vi "NF90 calibrator.vi"(9 "Ports":T1, 10 "channel index":i8) -> ()   [LabVIEW 2015]
doc: "Illustrates the simplest form of TCP data acquisition using a TCP data server.\n\n\nCreated by Monroe Weber-Shirk\nCornell University\nmw24@cornell.edu\nJanuary 2000"
uses:
  NF90 move.ctl
  Axis.ctl
  DAC apps/support/method.ctl
  DataServer/command cluster.ctl
  DataServer/command.ctl
  DAQ configuration/Sensor array.ctl
  DAQ configuration/channel identifier.ctl
  NF90 commands.ctl
  DAQ configuration/Sensor buffer command.ctl
panel:
  in  "Go to Start":bool
  in  "Save Data":bool
  in  "Save Calibration":bool
  in  "Calibrate":bool
  in  "Go Home":bool
  in  "Done":bool
  in  "Find Home":bool
  in  "Acceleration":u8=6 min=1 max=50 step=1
  in  "Speed":sgl=1.0 min=0 max=3 format="%.3f"
  out "sample time":dbl format="%.2f"
  out "Sample rate":dbl format="%.2f"
  out "Error":cluster{sgl[], dbl[]}[](graph)
  in  "polynomial order":i32=2 min=1 max=5 step=1
  out "Calibation data":cluster{sgl[], "Best Polynomial Fit":dbl[]}[](graph)
  in  "Number of locations":u8=5 min=2 step=1
  in  "Start position":sgl min=-1048575 max=1048575 format="%.2f"
  in  "delay after move":u32=1000
  in  "Final position":sgl=10.0 min=-1048575 max=1048575 format="%.2f"
  in  "data points to acquire":u32=1000 min=1
  in  "method":T3={"sampling interval"=0.1, "samples to average"=1, "data interval"=0.0, "stream data"=FALSE, "file path"=refnum, "command"={"command"=enum."Idle", "start time (ms)"=0, "Channel Indices"=[], "Scans per Sample"=1}} {"command"."Scans per Sample" min=1; "data interval" format="%.2f"; "samples to average" min=1 step=1; "sampling interval" format="%.2f"}
  in  "move":T6={"axis"=enum."Z", "Increment"=0.0, "Speed"=1.0, "Acceleration"=1} {"Speed" min=0 format="%.3f"; "Acceleration" min=1 max=50 step=1; "Increment" format="%.3f"}
  in  "Home offset from limit switch":sgl min=-1048575 max=1048575 format="%.2f"
  out "Position":sgl(slide) min=0 max=6 step=-1 scale=0.0..1.0 scale format="%.2f"
  in  "serial port":refnum<visa-resource-name>="COM1"
  in  "stop":bool
  # "cm"
  # "cm/s"
  # "cm/s^2"
  # "cm"
  # "cm"
  # "Hz"
  # "s"
  # "ms"
  # "This code most likely doesn't work yet!"
  # "s"
  # "s"
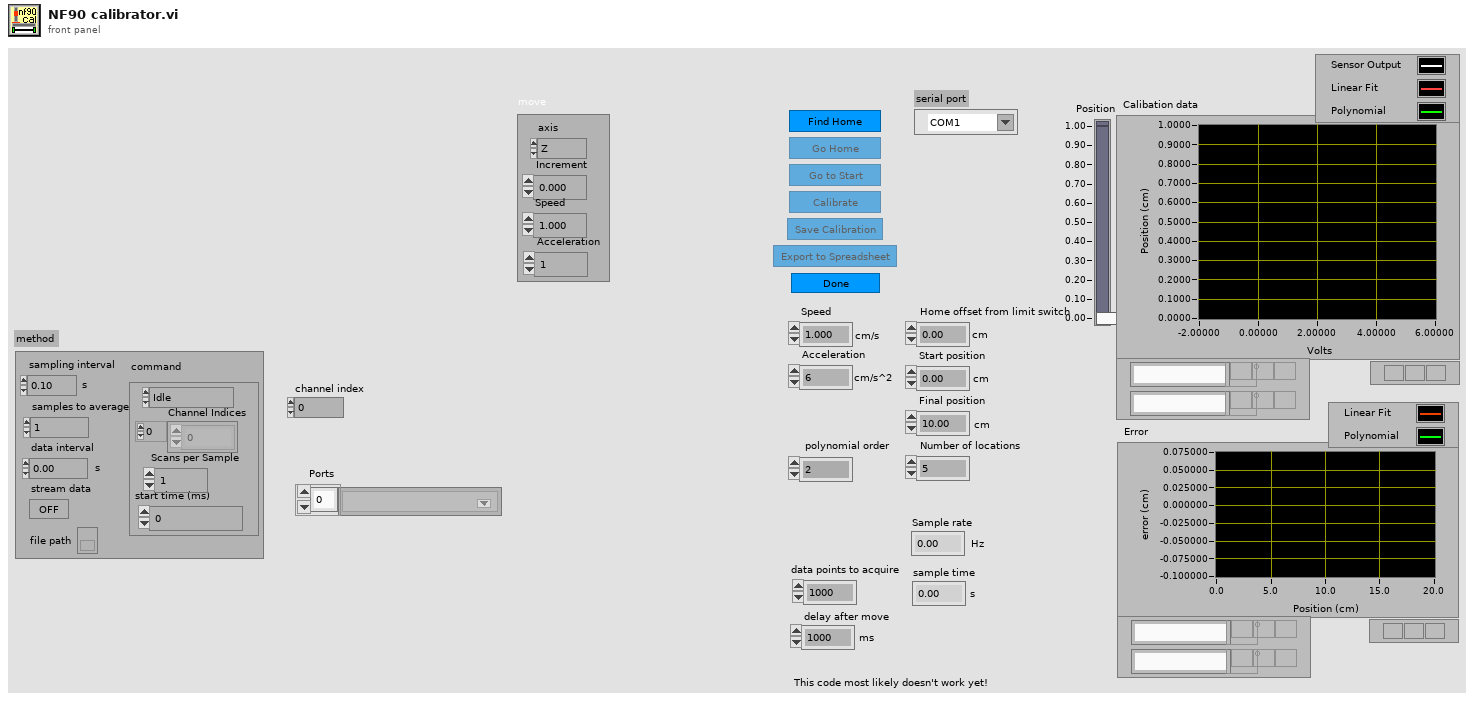
[diagram p1: front panel]
types:
  T1 = typedef "Sensor array.ctl" = T2[]
  T2 = typedef "channel identifier.ctl" = u16
  T3 = typedef "method.ctl" = cluster{"sampling interval":sgl, "samples to average":u32, "data interval":sgl, "stream data":bool, "file path":refnum<file>, "command":T4}
  T4 = typedef "command cluster.ctl" = cluster{"command":T5, "start time (ms)":u32, "Channel Indices":i32[], "Scans per Sample":i32}
  T5 = typedef "command.ctl" = enum16{"Idle", "Send Data", "Send 1 Scan", "Logoff"}
  T6 = typedef "NF90 move.ctl" = cluster{"axis":T7, "Increment":sgl, "Speed":sgl, "Acceleration":u8}
  T7 = typedef "Axis.ctl" = enum16{"X", "Y", "Z"}
  T8 = typedef "NF90 commands.ctl" = enum16{"Index", "Speed", "Acceleration", "Backlash", "Quit", "Run", "Null indexes", "Verify status", "Clear program", "Computer Control", "Go", "Put Controller on Hold", "Position"}
  T9 = typedef "Sensor buffer command.ctl" = enum16{"read average", "read recent", "read all", "write", "set buffer size", "Read channel config", "Write channel config", "clear"}
  T10 = typedef "Channel config.ctl" = cluster{"Channel Indices":T2[], "AI Max voltage":dbl[], "Calibration matrix":T11}
  T11 = typedef "calib array.ctl" = T12[]
  T12 = typedef "conversion.ctl" = cluster{"conversion matrix":sgl[][], "units":string, "name":string, "scale type":T13, "offset (volts)":dbl, "second channel":i8, "correspondence table":T14, "offset (physical units)":dbl, "pH scale":T15, "D.O.":T16, "Photometer data":T17}
  T13 = typedef "scale type.ctl" = enum16{"Volts", "Polynomial", "Correspondence Table", "pH", "Dissolved Oxygen", "Quadratic", "Photometer"}
  T14 = typedef "correspondence table.ctl" = cluster{"physical units":dbl, "volts":dbl}[]
  T15 = typedef "pH scale.ctl" = cluster{"Buffers":cluster{"Buffer":dbl, "Calibrated":bool, "V/T":dbl}[], "Temperature":dbl}
  T16 = typedef "DO scale.ctl" = cluster{"Temperature":dbl, "K":dbl, "barometric pressure":dbl}
  T17 = typedef "Photometer calibration data.ctl" = cluster{"Dark Voltage":dbl, "Blank Voltage":dbl, "Standards":cluster{"Concentration":dbl, "Voltage":dbl}[]}
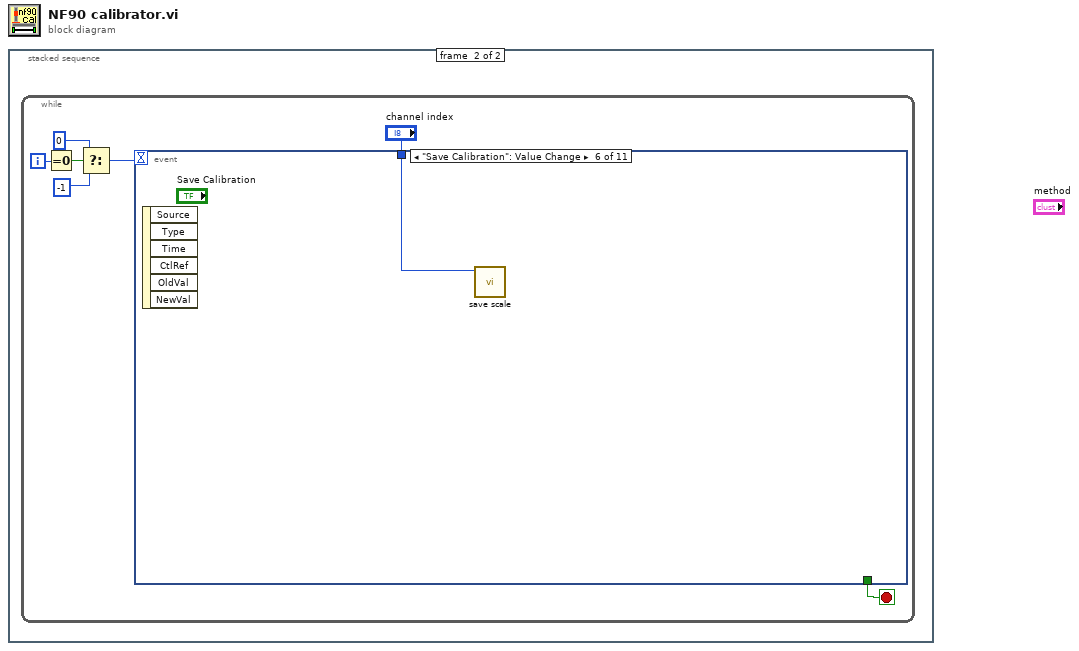
[diagram p0: block diagram]
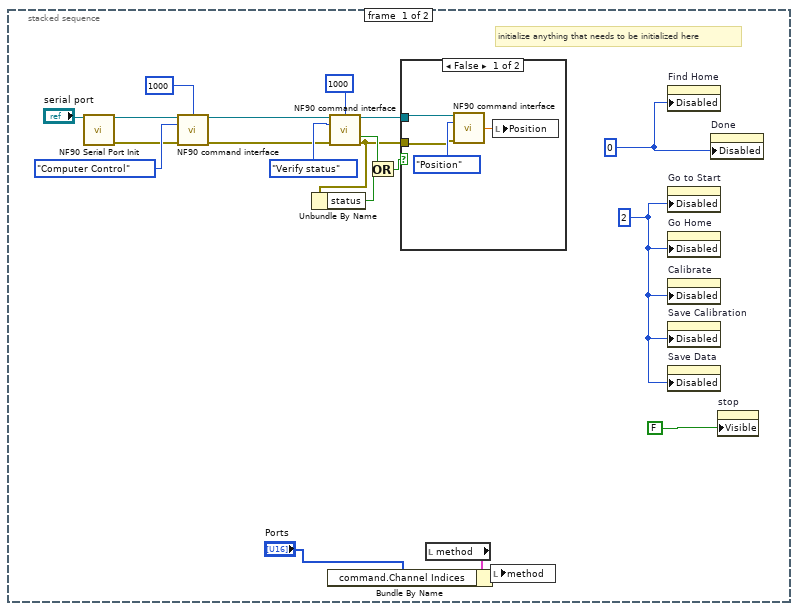
[diagram p2: hidden frame]
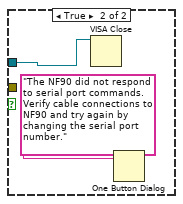
[diagram p3: hidden frame]
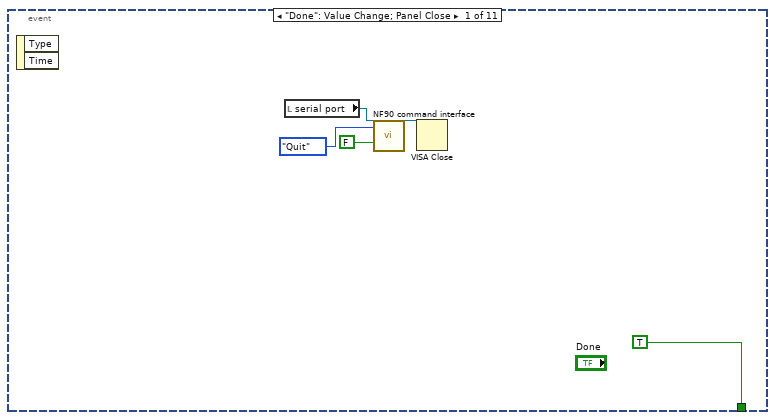
[diagram p4: hidden frame]
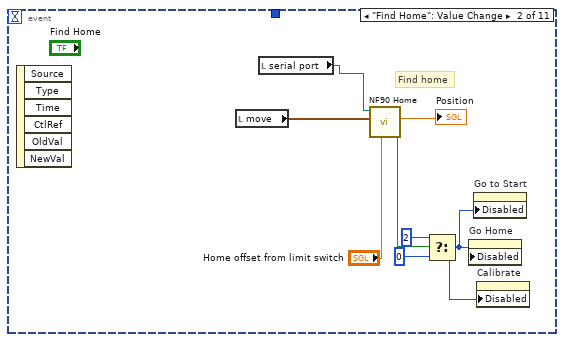
[diagram p5: hidden frame]
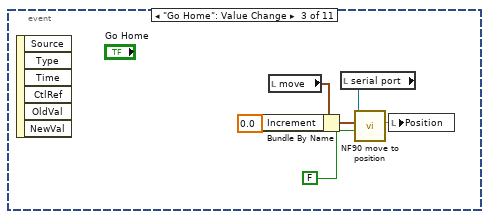
[diagram p6: hidden frame]
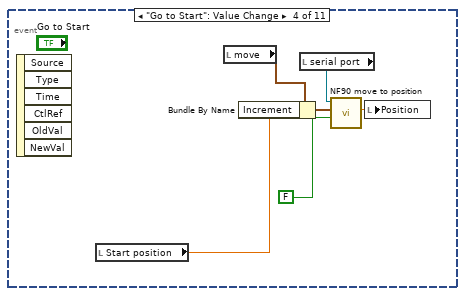
[diagram p7: hidden frame]
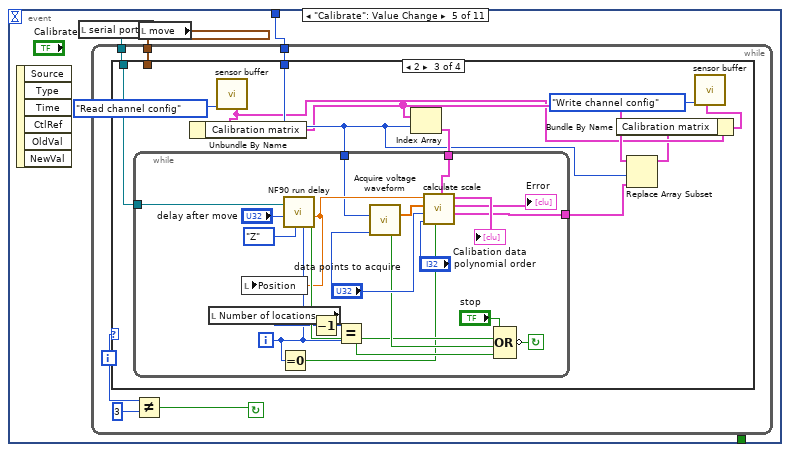
[diagram p8: hidden frame]
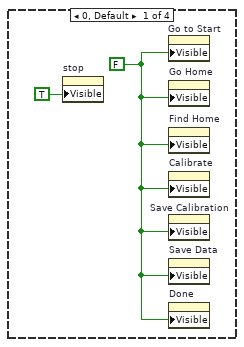
[diagram p9: hidden frame]
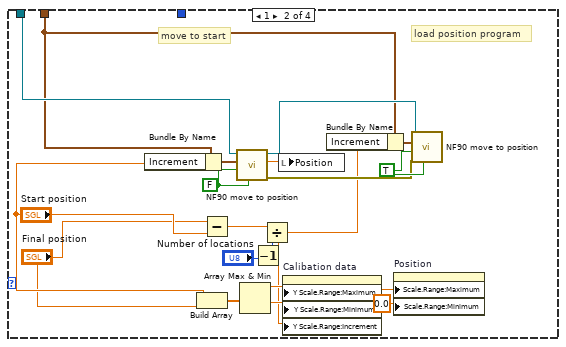
[diagram p10: hidden frame]
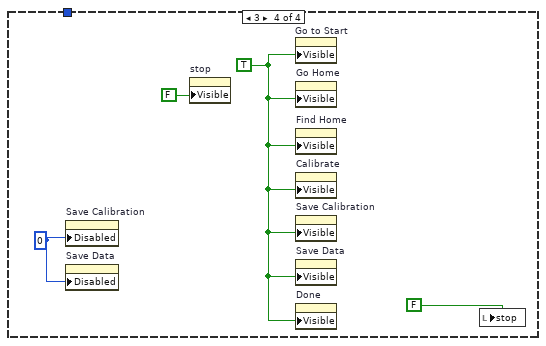
[diagram p11: hidden frame]
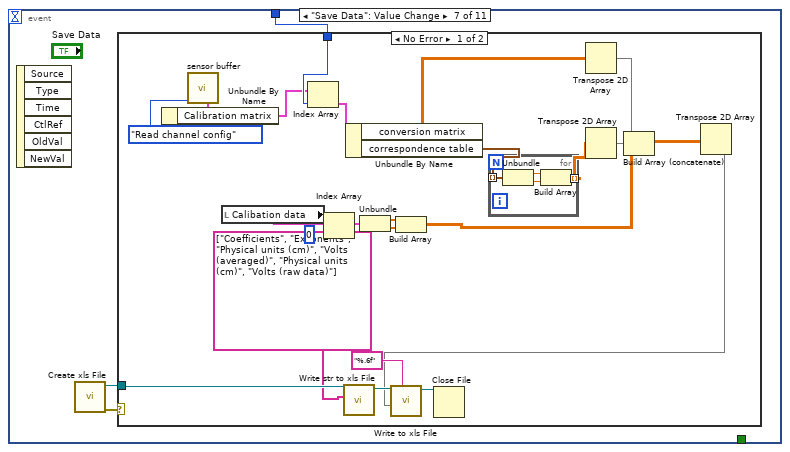
[diagram p12: hidden frame]
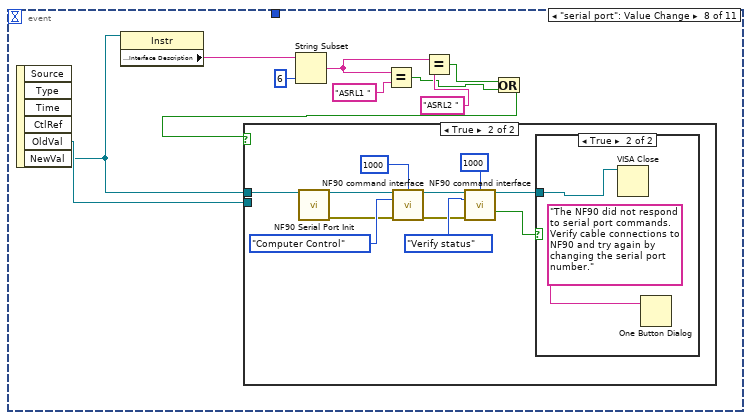
[diagram p14: hidden frame]
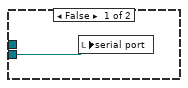
[diagram p15: hidden frame]
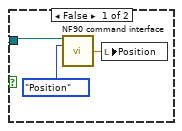
[diagram p16: hidden frame]
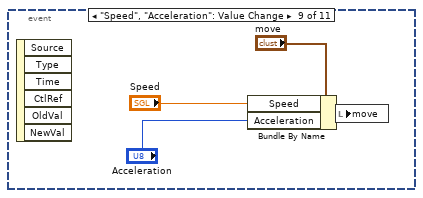
[diagram p17: hidden frame]
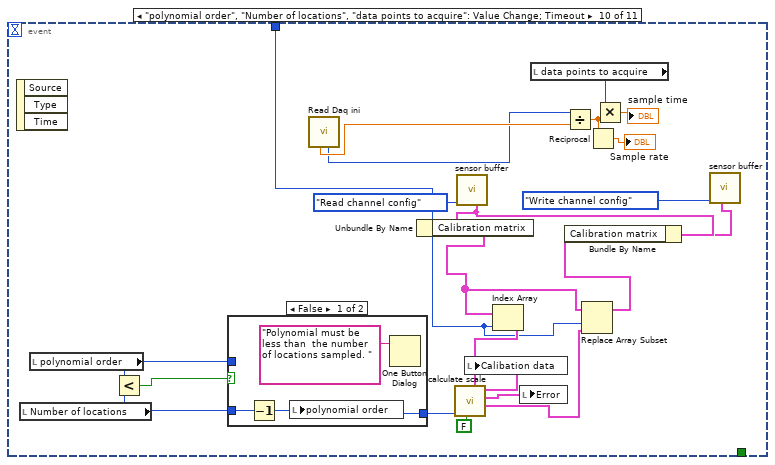
[diagram p18: hidden frame]
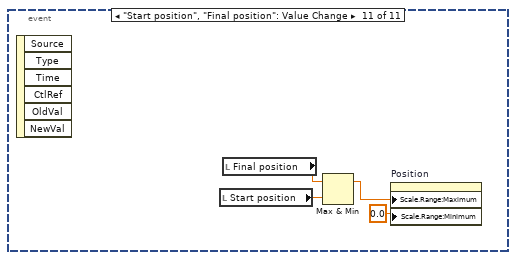
[diagram p20: hidden frame]
diagram:
  n1 = stacked-sequence {
    frame #0 {
      w10 = u8 2 ("Disabled")
      w9 = u8 0 ("Disabled")
      # "initialize anything that needs to be initialized here"
      n2 = call "NF90 Serial Port Init.vi"("port number"="serial port") -> ("port number"=w20:refnum<visa-resource-name>, "error out"=w7:errorcluster)  [unwired: 13 in]
      n3 = call "NF90 command interface.vi"("port number in"=w20, "time out (ms)"=u32 1000, "commands"=NF90_commands."Computer Control", "Error In"=w7) -> ("port number out"=w16:refnum<visa-resource-name>, "Error Out"=w6:errorcluster)  [unwired: 7 in, 3 out]
      n4 = call "NF90 command interface.vi"("port number in"=w16, "time out (ms)"=u32 1000, "commands"=NF90_commands."Verify status", "Error In"=w6) -> ("port number out"=w15:refnum<visa-resource-name>, "timed out"=w4:bool, "Error Out"=w2:errorcluster)  [unwired: 7 in, 2 out]
      n5 = Unbundle By Name(w2) -> ("status"=w5:bool)
      n6 = Or(x=w4, y=w5) -> (x .or. y?=w3:bool)
      n7 = case shown="False" w3 {
        tunnel: w15 -> [w22 w25]
        tunnel: w2 -> [w21 _]
        frame False {
          n8 = call "NF90 command interface.vi"("port number in"=w22, "commands"=NF90_commands."Position", "Error In"=w21) -> ("Position"=w23:sgl)  [unwired: 8 in, 4 out]
          n9 = local write "Position"(w23) -> ()
        }
        frame True {
          n10 = VISA Close(VISA resource name=w25) -> ()  [unwired: 1 in, 1 out]
          n11 = One Button Dialog(message="The NF90 did not respond to serial port commands. Verify cable connections to NF90 and try again by changing the serial port number.") -> ()  [unwired: 1 in, 1 out]
        }
      }
      n12 = local read "method"() -> (w12:T3)
      n13 = Bundle By Name(cluster=w12, "command.Channel Indices"="Ports") -> (w11:T3)
      n14 = local write "method"(w11) -> ()
      n15 = property on="Find Home" class="Bool"("Disabled"=w9) -> ()  [unwired: 2 in, 2 out]
      n16 = property on="Go to Start" class="Bool"("Disabled"=w10) -> ()  [unwired: 2 in, 2 out]
      n17 = property on="Go Home" class="Bool"("Disabled"=w10) -> ()  [unwired: 2 in, 2 out]
      n18 = property on="Calibrate" class="Bool"("Disabled"=w10) -> ()  [unwired: 2 in, 2 out]
      n19 = property on="Save Calibration" class="Bool"("Disabled"=w10) -> ()  [unwired: 2 in, 2 out]
      n20 = property on="Save Data" class="Bool"("Disabled"=w10) -> ()  [unwired: 2 in, 2 out]
      n21 = property on="Done" class="Bool"("Disabled"=w9) -> ()  [unwired: 2 in, 2 out]
      n22 = property on="stop" class="Bool (strict)"("Visible"=FALSE) -> ()  [unwired: 2 in, 2 out]
    }
    frame #1 {
      n23 = while {
        i -> [w31]
        stop <- w32 stop-if-true
        n24 = Equal To 0?(x=w31) -> (x = 0?=w30:bool)
        n25 = Select(t=0, s=w30, f=-1) -> (s? t:f=w27:i32)
        n26 = event shown="[5] \"Save Calibration\": Value Change" {
          selector: _ -> [_ _ _ _ _ _ _ _ _ _ _]
          dyn-events: _ -> [_ _ _ _ _ _ _ _ _ _ _]
          timeout: w27 -> [_ _ _ _ _ _ _ _ _ _ _]
          tunnel: "channel index" -> [_ _ _ _ w61 w124 w125 _ _ w194 _]
          tunnel: [TRUE _ _ _ _ _ _ _ _ _ _] -> w32
          event "Done": Value Change; Panel Close {
            n27 = event-data() -> ()  [unwired: 1 in, 2 out]
            n28 = local read "serial port"() -> (w35:refnum<visa-resource-name>)
            n29 = call "NF90 command interface.vi"("port number in"=w35, "commands"=NF90_commands."Quit", "enable?"=FALSE) -> ("port number out"=w38:refnum<visa-resource-name>)  [unwired: 8 in, 4 out]
            n30 = VISA Close(VISA resource name=w38) -> ()  [unwired: 1 in, 1 out]
          }
          event "Find Home": Value Change {
            # "Find home"
            n31 = event-data() -> ()  [unwired: 1 in, 6 out]
            n32 = local read "move"() -> (w41:T6)
            n33 = local read "serial port"() -> (w40:refnum<visa-resource-name>)
            n34 = call "NF90 Home.vi"("Index offset from switch"="Home offset from limit switch", "move"=w41, "port number in"=w40) -> ("killed"=w44:bool, "position"=→"Position":dbl)  [unwired: 4 in, 2 out]
            n35 = Select(t=2, s=w44, f=0) -> (s? t:f=w39:i32)
            n36 = property on="Go Home" class="Bool"("Disabled"=w39) -> ()  [unwired: 2 in, 2 out]
            n37 = property on="Go to Start" class="Bool"("Disabled"=w39) -> ()  [unwired: 2 in, 2 out]
            n38 = property on="Calibrate" class="Bool"("Disabled"=w39) -> ()  [unwired: 2 in, 2 out]
          }
          event "Go Home": Value Change {
            n39 = event-data() -> ()  [unwired: 1 in, 6 out]
            n40 = local read "move"() -> (w47:T6)
            n41 = Bundle By Name(cluster=w47, "Increment"=sgl 0.0 ("Bundle Element")) -> (w49:T6)
            n42 = local read "serial port"() -> (w48:refnum<visa-resource-name>)
            n43 = call "NF90 move to position.vi"("move type (abs = False)"=FALSE ("move type (abs = true)"), "move"=w49, "port number in"=w48) -> ("Position out"=w52:sgl)  [unwired: 4 in, 3 out]
            n44 = local write "Position"(w52) -> ()
          }
          event "Go to Start": Value Change {
            n45 = event-data() -> ()  [unwired: 1 in, 6 out]
            n46 = local read "Start position"() -> (w58:sgl)
            n47 = local read "move"() -> (w53:T6)
            n48 = Bundle By Name(cluster=w53, "Increment"=w58) -> (w55:T6)
            n49 = local read "serial port"() -> (w54:refnum<visa-resource-name>)
            n50 = call "NF90 move to position.vi"("move type (abs = False)"=FALSE ("move type (abs = true)"), "move"=w55, "port number in"=w54) -> ("Position out"=w57:sgl)  [unwired: 4 in, 3 out]
            n51 = local write "Position"(w57) -> ()
          }
          event "Calibrate": Value Change {
            n52 = event-data() -> ()  [unwired: 1 in, 6 out]
            n53 = local read "serial port"() -> (w60:refnum<visa-resource-name>)
            n54 = local read "move"() -> (w59:T6)
            n55 = while {
              tunnel: w60 -> [w65]
              tunnel: w59 -> [w66]
              tunnel: w61 -> [w62]
              i -> [w67]
              stop <- w63 continue-if-true
              n56 = case shown="2" w67 {
                tunnel: w66 -> [_ w81 _ _]
                tunnel: w65 -> [_ w87 w98 _]
                tunnel: w62 -> [_ _ w95 _]
                frame 0, Default {
                  w69 = FALSE ("Visible")
                  n57 = property on="stop" class="Bool (strict)"("Visible"=TRUE) -> ()  [unwired: 2 in, 2 out]
                  n58 = property on="Go to Start" class="Bool"("Visible"=w69) -> ()  [unwired: 2 in, 2 out]
                  n59 = property on="Go Home" class="Bool"("Visible"=w69) -> ()  [unwired: 2 in, 2 out]
                  n60 = property on="Find Home" class="Bool"("Visible"=w69) -> ()  [unwired: 2 in, 2 out]
                  n61 = property on="Calibrate" class="Bool"("Visible"=w69) -> ()  [unwired: 2 in, 2 out]
                  n62 = property on="Save Calibration" class="Bool"("Visible"=w69) -> ()  [unwired: 2 in, 2 out]
                  n63 = property on="Save Data" class="Bool"("Visible"=w69) -> ()  [unwired: 2 in, 2 out]
                  n64 = property on="Done" class="Bool"("Visible"=w69) -> ()  [unwired: 2 in, 2 out]
                }
                frame 1 {
                  w80 = FALSE ("move type (abs = true)")
                  w79 = TRUE ("move type (abs = False)")
                  # "move to start"
                  # "load position program"
                  n65 = Bundle By Name(cluster=w81, "Increment"="Start position") -> (w88:T6)
                  n66 = Build Array("Start position", "Final position") -> (w74:sgl[])
                  n67 = Subtract(x="Final position", y="Start position") -> (x-y=w84:sgl)
                  n68 = call "NF90 move to position.vi"("program (Run=False)"=w80, "move type (abs = False)"=w80, "move"=w88, "port number in"=w87) -> ("Error Out"=w78:errorcluster, "Position out"=w77:sgl, "port number out"=w86:refnum<visa-resource-name>)  [unwired: 3 in, 1 out]
                  n69 = Array Max & Min(array=w74) -> (max value=w73:sgl, min value=w72:sgl)  [unwired: 2 out]
                  n70 = Decrement(x="Number of locations") -> (x-1=w83:u8)
                  n71 = Divide(x=w84, y=w83) -> (x/y=w71:sgl)
                  n72 = local write "Position"(w77) -> ()
                  n73 = property on="Calibation data" class="XYGraph (strict)"("Y Scale.Range:Maximum"=w73, "Y Scale.Range:Minimum"=w72, "Y Scale.Range:Increment"=w71) -> ()  [unwired: 2 in, 2 out]
                  n74 = Bundle By Name(cluster=w81, "Increment"=w71) -> (w82:T6)
                  n75 = property on="Position" class="Slide (strict)"("Scale.Range:Maximum"=w73, "Scale.Range:Minimum"=0.0) -> ()  [unwired: 2 in, 2 out]
                  n76 = call "NF90 move to position.vi"("program (Run=False)"=w79, "Error In"=w78, "move type (abs = False)"=w79, "move"=w82, "port number in"=w86) -> ()  [unwired: 2 in, 4 out]
                }
                frame 2 {
                  n77 = call "sensor buffer.vi"("command"=Sensor_buffer_command."Read channel config") -> ("Channel Config out"=w91:T10)  [unwired: 6 in, 4 out]
                  n78 = Unbundle By Name(w91) -> ("Calibration matrix"=w93:T11)
                  n79 = Index Array(array=w93, index=w95) -> (element=w97:T12)
                  n80 = while {
                    tunnel: [w106] -> w96
                    tunnel: w98 -> [w119]
                    tunnel: w95 -> [w100]
                    tunnel: w97 -> [w99]
                    i -> [w102]
                    stop <- w116 continue-if-true
                    n81 = local read "Number of locations"() -> (w112:u8)
                    n82 = Equal To 0?(x=w102) -> (x = 0?=w101:bool)
                    n83 = call "NF90 run delay.vi"("i"=w102, "axis"=Axis."Z", "delay (ms)"="delay after move", "port number"=w119) -> ("Position"=w108:sgl, "killed"=w114:bool)  [unwired: 4 in, 2 out]
                    n84 = local write "Position"(w108) -> ()
                    n85 = Decrement(x=w112) -> (x-1=w105:u8)
                    n86 = Equal?(x=w105, y=w102) -> (x = y?=w111:bool)
                    n87 = call "Acquire voltage waveform.vi"("channel index"=w100, "data points to acquire"="data points to acquire") -> ("channel data array"=w109:sgl[], "canceled"=w115:bool)  [unwired: 10 in, 2 out]
                    n88 = call "calculate scale.vi"("Scaling in"=w99, "reset"=w101, "polynomial order"="polynomial order", "data points to acquire"="data points to acquire", "volts array"=w109, "Position"=w108) -> ("Scaling out"=w106:T12, "error graph"=→"Error":cluster{"X array":sgl[], "Y array":dbl[]}[], "Output Graph"=→"Calibation data":cluster{"X array":sgl[], "Y array":dbl[]}[])  [unwired: 2 in]
                    n89 = Compound Arithmetic op=OR("stop", w114, w115, w111) -> (invert w116:bool)
                  }
                  n90 = Replace Array Subset(array=w93, new element=w96, index=w95) -> (w89:T11)
                  n91 = Bundle By Name(cluster=w91, "Calibration matrix"=w89) -> (w90:T10)
                  n92 = call "sensor buffer.vi"("Channel Config"=w90, "command"=Sensor_buffer_command."Write channel config") -> ()  [unwired: 5 in, 5 out]
                }
                frame 3 {
                  w122 = TRUE ("Visible")
                  w120 = u8 0 ("Disabled")
                  n93 = property on="Save Calibration" class="Bool"("Disabled"=w120) -> ()  [unwired: 2 in, 2 out]
                  n94 = property on="Save Data" class="Bool"("Disabled"=w120) -> ()  [unwired: 2 in, 2 out]
                  n95 = property on="stop" class="Bool (strict)"("Visible"=FALSE) -> ()  [unwired: 2 in, 2 out]
                  n96 = property on="Go to Start" class="Bool"("Visible"=w122) -> ()  [unwired: 2 in, 2 out]
                  n97 = property on="Go Home" class="Bool"("Visible"=w122) -> ()  [unwired: 2 in, 2 out]
                  n98 = property on="Find Home" class="Bool"("Visible"=w122) -> ()  [unwired: 2 in, 2 out]
                  n99 = property on="Calibrate" class="Bool"("Visible"=w122) -> ()  [unwired: 2 in, 2 out]
                  n100 = property on="Save Calibration" class="Bool"("Visible"=w122) -> ()  [unwired: 2 in, 2 out]
                  n101 = property on="Save Data" class="Bool"("Visible"=w122) -> ()  [unwired: 2 in, 2 out]
                  n102 = property on="Done" class="Bool"("Visible"=w122) -> ()  [unwired: 2 in, 2 out]
                  n103 = local write "stop"(FALSE ("Visible")) -> ()
                }
              }
              n104 = Not Equal?(x=w67, y=3) -> (x != y?=w63:bool)
            }
          }
          event "Save Calibration": Value Change {
            n105 = event-data() -> ()  [unwired: 1 in, 6 out]
            n106 = call "save scale.vi"("Index"=w124) -> ()  [unwired: 9 in, 1 out]
          }
          event "Save Data": Value Change {
            n107 = event-data() -> ()  [unwired: 1 in, 6 out]
            n108 = call "Create xls File.vi"() -> ("error out"=w127:errorcluster, "refnum"=w126:refnum<file>)  [unwired: 4 in, 2 out]
            n109 = case shown="No Error" w127 {
              tunnel: w126 -> [w134 _]
              tunnel: w125 -> [w133 _]
              frame No Error {
                n110 = call "sensor buffer.vi"("command"=Sensor_buffer_command."Read channel config") -> ("Channel Config out"=w129:T10)  [unwired: 6 in, 4 out]
                n111 = Unbundle By Name(w129) -> ("Calibration matrix"=w128:T11)
                n112 = local read "Calibation data"() -> (w138:cluster{sgl[], "Best Polynomial Fit":dbl[]}[])
                n113 = Index Array(array=w128, index=w133) -> (element=w132:T12)
                n114 = Index Array(array=w138, index=0 ("Index")) -> (element=w137:cluster{sgl[], "Best Polynomial Fit":dbl[]})
                n115 = call "Write str to xls File.vi"("1D data"=string[] ["Coefficients", "Exponents", "Physical units (cm)", "Volts (averaged)", "Physical units (cm)", "Volts (raw data)"], "refnum"=w134) -> ("dup refnum"=w150:refnum<file>)  [unwired: 8 in, 1 out]
                n116 = Unbundle By Name(w132) -> ("conversion matrix"=w145:sgl[][], "correspondence table"=w148:T14)
                n117 = Unbundle(w137) -> (w140:sgl[], "Best Polynomial Fit"=w139:dbl[])
                n118 = Build Array(w140, w139) -> (w135:dbl[][])
                n119 = for {
                  tunnel: w148 -> [w154] mode=indexing
                  tunnel: [w151] -> w147 mode=indexing
                  n120 = Unbundle(w154) -> ("physical units"=w153:dbl, "volts"=w152:dbl)
                  n121 = Build Array(w153, w152) -> (w151:dbl[])
                }
                n122 = Transpose 2D Array(2D array=w145) -> (transposed array=w143:sgl[][])
                n123 = Transpose 2D Array(2D array=w147) -> (transposed array=w142:dbl[][])
                n124 = Build Array (concatenate)(w143, w142, w135) -> (w146:dbl[][])
                n125 = Transpose 2D Array(2D array=w146) -> (transposed array=w141:dbl[][])
                n126 = call "Write to xls File.vi"("format (%.3f)"="%.6f", "2D data"=w141, "refnum"=w150) -> ("dup refnum"=w149:refnum<file>)  [unwired: 7 in, 1 out]
                n127 = Close File(refnum=w149) -> ()  [unwired: 1 in, 2 out]
              }
              frame Error {
              }
            }
          }
          event "serial port": Value Change {
            n128 = event-data() -> ("OldVal"=w163:refnum<visa-resource-name>, "NewVal"=w155:refnum<visa-resource-name>)  [unwired: 1 in, 4 out]
            n129 = property class="Instr"(reference=w155) -> ("Interface Information:Interface Description"=w158:string)  [unwired: 1 in, 2 out]
            n130 = String Subset(string=w158, length (rest)=6 ("length (rest)")) -> (substring=w157:string)  [unwired: 1 in]
            n131 = Equal?(x=w157, y="ASRL1 ") -> (x = y?=w160:bool)
            n132 = Equal?(x=w157, y="ASRL2 ") -> (x = y?=w161:bool)
            n133 = Or(x=w161, y=w160) -> (x .or. y?=w159:bool)
            n134 = case shown="True" w159 {
              tunnel: w155 -> [_ w166]
              tunnel: w163 -> [w165 _]
              frame False {
                n135 = local write "serial port"(w165) -> ()
              }
              frame True {
                n136 = call "NF90 Serial Port Init.vi"("port number"=w166) -> ("port number"=w176:refnum<visa-resource-name>, "error out"=w168:errorcluster)  [unwired: 13 in]
                n137 = call "NF90 command interface.vi"("port number in"=w176, "time out (ms)"=u32 1000, "commands"=NF90_commands."Computer Control", "Error In"=w168) -> ("port number out"=w173:refnum<visa-resource-name>, "Error Out"=w167:errorcluster)  [unwired: 7 in, 3 out]
                n138 = call "NF90 command interface.vi"("port number in"=w173, "time out (ms)"=u32 1000, "commands"=NF90_commands."Verify status", "Error In"=w167) -> ("port number out"=w172:refnum<visa-resource-name>, "timed out"=w169:bool)  [unwired: 7 in, 3 out]
                n139 = case shown="True" w169 {
                  tunnel: w172 -> [w177 w180]
                  frame False {
                    n140 = call "NF90 command interface.vi"("port number in"=w177, "commands"=NF90_commands."Position") -> ("Position"=w178:sgl)  [unwired: 9 in, 4 out]
                    n141 = local write "Position"(w178) -> ()
                  }
                  frame True {
                    n142 = VISA Close(VISA resource name=w180) -> ()  [unwired: 1 in, 1 out]
                    n143 = One Button Dialog(message="The NF90 did not respond to serial port commands. Verify cable connections to NF90 and try again by changing the serial port number.") -> ()  [unwired: 1 in, 1 out]
                  }
                }
              }
            }
          }
          event "Speed", "Acceleration": Value Change {
            n144 = event-data() -> ()  [unwired: 1 in, 6 out]
            n145 = Bundle By Name(cluster="move", "Speed"="Speed", "Acceleration"="Acceleration") -> (w182:T6)
            n146 = local write "move"(w182) -> ()
          }
          event "polynomial order", "Number of locations", "data points to acquire": Value Change; Timeout {
            n147 = event-data() -> ()  [unwired: 1 in, 3 out]
            n148 = local read "Number of locations"() -> (w197:u8)
            n149 = local read "polynomial order"() -> (w195:i32)
            n150 = Less?(x=w195, y=w197) -> (x < y?=w196:bool)
            n151 = case shown="False" w196 {
              tunnel: w197 -> [w210 _]
              tunnel: [w208 w211] -> w198
              tunnel: w195 -> [_ w211]
              frame False {
                n152 = Decrement(x=w210) -> (x-1=w208:u8)
                n153 = local write "polynomial order"(w208) -> ()
                n154 = One Button Dialog(message="Polynomial must be less than  the number of locations sampled. ") -> ()  [unwired: 1 in, 1 out]
              }
              frame True {
              }
            }
            n155 = call "Read Daq ini.vi"() -> ("samples per read"=w186:i32, "Data rate (hz)"=w187:dbl)  [unwired: 3 in, 7 out]
            n156 = call "sensor buffer.vi"("command"=Sensor_buffer_command."Read channel config") -> ("Channel Config out"=w189:T10)  [unwired: 6 in, 4 out]
            n157 = Unbundle By Name(w189) -> ("Calibration matrix"=w191:T11)
            n158 = Index Array(array=w191, index=w194) -> (element=w202:T12)
            n159 = call "calculate scale.vi"("Scaling in"=w202, "reset"=FALSE, "polynomial order"=w198) -> ("Scaling out"=w203:T12, "error graph"=w200:cluster{"X array":sgl[], "Y array":dbl[]}[], "Output Graph"=w199:cluster{"X array":sgl[], "Y array":dbl[]}[])  [unwired: 5 in]
            n160 = local write "Calibation data"(w199) -> ()
            n161 = local write "Error"(w200) -> ()
            n162 = local read "data points to acquire"() -> (w204:u32)
            n163 = Divide(x=w186, y=w187) -> (x/y=w206:dbl)
            n164 = Replace Array Subset(array=w191, new element=w203, index=w194) -> (w190:T11)
            n165 = Bundle By Name(cluster=w189, "Calibration matrix"=w190) -> (w188:T10)
            n166 = Reciprocal(x=w206) -> (1/x=→"Sample rate":dbl)
            n167 = Multiply(x=w204, y=w206) -> (x*y=→"sample time":dbl)
            n168 = call "sensor buffer.vi"("Channel Config"=w188, "command"=Sensor_buffer_command."Write channel config") -> ()  [unwired: 5 in, 5 out]
          }
          event "Start position", "Final position": Value Change {
            n169 = event-data() -> ()  [unwired: 1 in, 6 out]
            n170 = local read "Start position"() -> (w214:sgl)
            n171 = local read "Final position"() -> (w215:sgl)
            n172 = Max & Min(x=w215, y=w214) -> (max(x,y)=w213:sgl)  [unwired: 1 out]
            n173 = property on="Position" class="Slide (strict)"("Scale.Range:Maximum"=w213, "Scale.Range:Minimum"=0.0) -> ()  [unwired: 2 in, 2 out]
          }
        }
      }
    }
  }
